vi "Sensor.vi"() -> (2 "camera mode vision":T1={"type"="heartbeat", "message"="{}"})   [LabVIEW 2016, in "Vision Server.lvclass"]
uses:
  Vision Server.lvclass
  typedef/Message Type.ctl
panel:
  in  "define":T1={"type"="sensor", "message"="{}"}
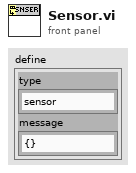
[diagram p1: front panel]
types:
  T1 = typedef "Vision Server.lvclass/Message Type.ctl" = cluster{"type":string, "message":string}
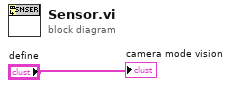
[diagram p0: block diagram]
diagram:
  "camera mode vision" <- "define"
